vi "Raise Resume Event.vi"(8 "error in (no error)":errorcluster, 9 "Send Resume":bool=TRUE, 10 "Raiser Id":string, 11 "Raiser Name":string) -> (0 "error out":errorcluster)   [LabVIEW 2023, in "HAF.lvlib"]
doc: "Helper member to raise a Resume Event. It is always sent as high priority."
uses:
  HAF.lvlib
  Event Data.ctl
  <vilib>/event_ctls.llb/usereventprio.ctl
  Resume Event.ctl
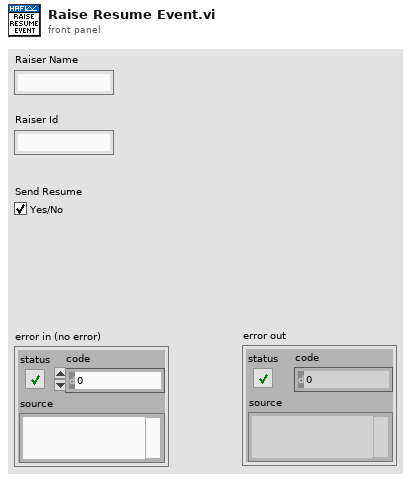
[diagram p1: front panel]
types:
  T1 = typedef "usereventprio.ctl" = enum32{"high priority", "normal priority"}
  T2 = typedef "HAF.lvlib/Event Data.ctl" = cluster{"Raiser Name":string, "Raiser Id":string}
  T3 = typedef "HAF.lvlib/Resume Event.ctl" = refnum<user-event>
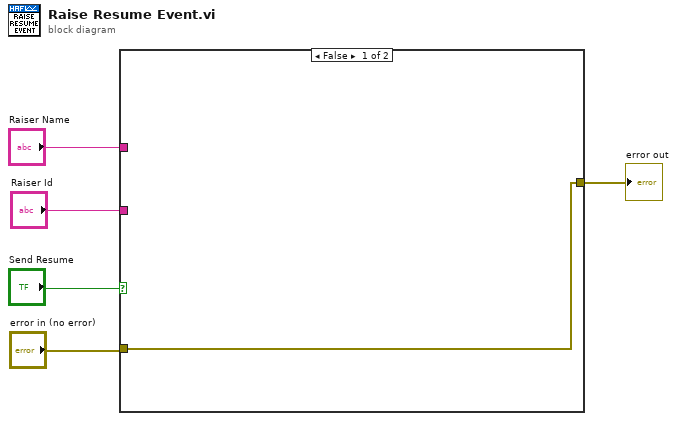
[diagram p0: block diagram]
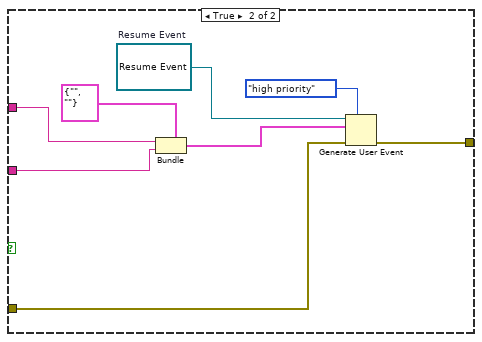
[diagram p2: hidden frame]
diagram:
  n1 = case shown="False" "Send Resume" {
    tunnel: "error in (no error)" -> [w6 w10]
    tunnel: "Raiser Name" -> [_ w13]
    tunnel: "Raiser Id" -> [_ w12]
    tunnel: [w6 w9] -> w1
    frame False {
    }
    frame True {
      w7 = T3 refnum  # Resume Event
      n2 = Bundle(cluster=T2 {"Raiser Name"="", "Raiser Id"=""} ("Event Data Structure"), "Raiser Name"=w13, "Raiser Id"=w12) -> (w11:T2)
      n3 = Generate User Event(priority (normal)=usereventprio."high priority", user event=w7, event data cluster=w11, error in=w10) -> (error out=w9:errorcluster)  [unwired: 1 out]
    }
  }
  "error out" <- w1
